vi "Alex_initialize.vi"() -> ()   [LabVIEW 2017]
panel:
  in  "VISA resource name":refnum<visa-resource-name>
  in  "Wait before read (0ms)":u32
  in  "Bytes to read (100)":u32=100
  out "Returned string":string
  in  "error in (no error) 2":errorcluster
  # "INITIALIZE"
  # "WRITE COMMAND AND READ"
  # "CLOSE"
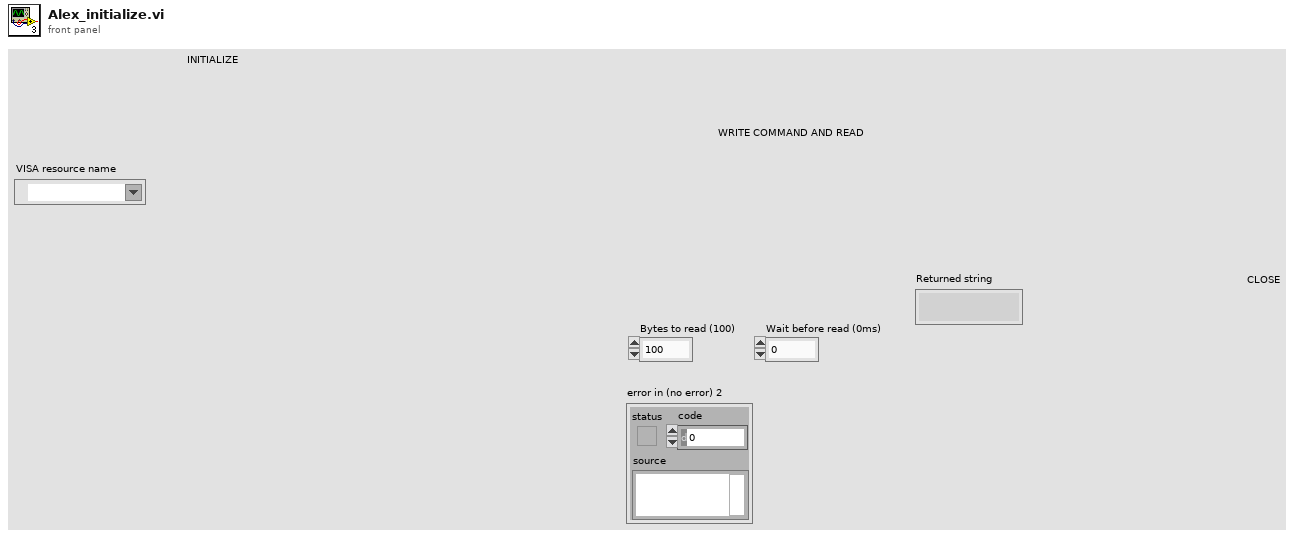
[diagram p1: front panel]
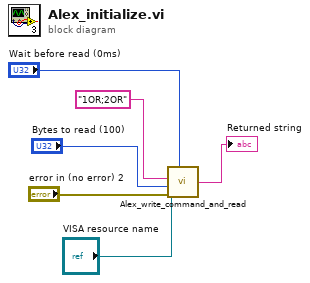
[diagram p0: block diagram]
diagram:
  n1 = call "Alex_write_command_and_read.vi"("VISA resource name"="VISA resource name", "Wait before read (0ms)"="Wait before read (0ms)", "Command"="1OR;2OR", "Bytes to read (100)"="Bytes to read (100)", "error in (no error)"="error in (no error) 2") -> ("Returned string"=→"Returned string":string)  [unwired: 3 in]
